vi "Construct.vi"(1 "y":dbl, 2 "x":dbl) -> (0 "Vec2 out":refnum<class "Vector2.lvclass">)   [LabVIEW 2022 SP3, in "Vector2.lvclass"]
uses:
  Vector2.lvclass
  Vector2.lvclass/Vector2.ctl
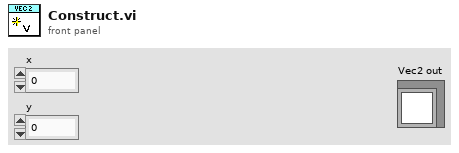
[diagram p1: front panel]
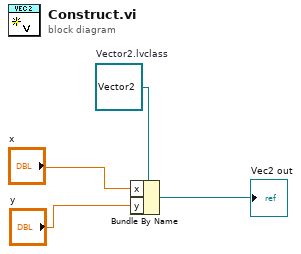
[diagram p0: block diagram]
diagram:
  w4 = refnum<class "Vector2.lvclass"> refnum  # Vector2.lvclass
  n1 = Bundle By Name(cluster=w4, "x"="x", "y"="y") -> (→"Vec2 out":refnum<class "Vector2.lvclass">)
